vi "Aliasing 1.vi"() -> ()   [LabVIEW 2016]
uses:
  <vilib>/measure/maresamp.llb/Resample Waveform (single shot).vi
  <vilib>/measure/NI_MABase.lvlib
  <vilib>/measure/NI_MAPro.lvlib
panel:
  in  "y-scale [V]":dbl=1.2
  in  "Resolution [Bit]":u8=12
  in  "Sample rate [1/s]":dbl=11.0 min=0.1 step=0.1 format="%.2p"
  in  "Range Volts]":dbl=1.0 format="%0.2p"
  out "Waveform Graph":waveform(dbl)[](graph)=[{"t0"=timestamp(0 s since 1904-01-01), "dt"=0.001, "Y"=array[2000 elements]}, {"t0"=timestamp(0 s since 1904-01-01), "dt"=0.09090909090909091, "Y"=[0.0, -0.5403941761363638, -0.9093128551136365, -0.9895241477272729, -0.755415482954545, -0.2815607244318157, 0.2815607244318157, 0.755415482954545, 0.9895241477272729, 0.9093128551136351, 0.5403941761363593, 0.0, -0.5403941761363593, -0.9093128551136379, -0.9895241477272729, -0.7554154829545403, -0.2815607244318157, 0.2815607244318157, 0.7554154829545497, 0.9895241477272729, 0.9093128551136322, 0.5403941761363593]}, {"t0"=timestamp(0 s since 1904-01-01), "dt"=0.0005, "Y"=array[4000 elements]}]
  in  "Stop":bool
  in  "Signal Type":T1(ring)
  in  "Duty cycle [%]":dbl=50.0
  in  "Phase [deg]":dbl format="%.2p"
  in  "Frequency [Hz]":dbl=10.0 min=0.0 max=100.0 step=0.1 format="%.2p"
  # "Original Wave"
  # "Sampled Wave"
  # "Sampling and Aliasing"
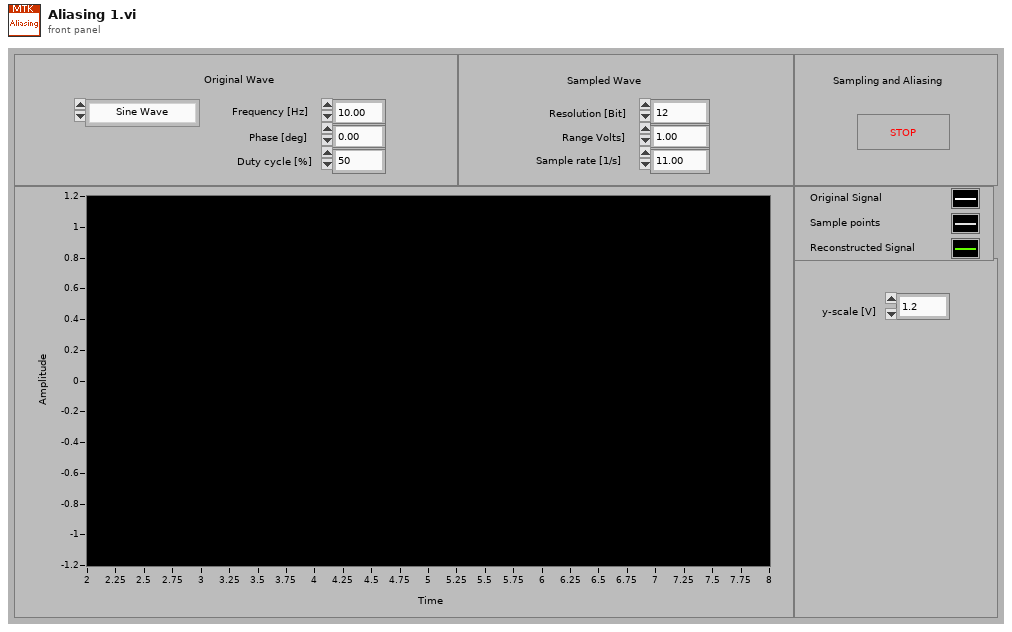
[diagram p1: front panel]
types:
  T1 = enum16{"Sine Wave", "Triangle Wave", "Square Wave", "Sawtooth Wave"}
  T2 = cluster{"Sample rate [1/s]":dbl, "No. of samples":dbl}
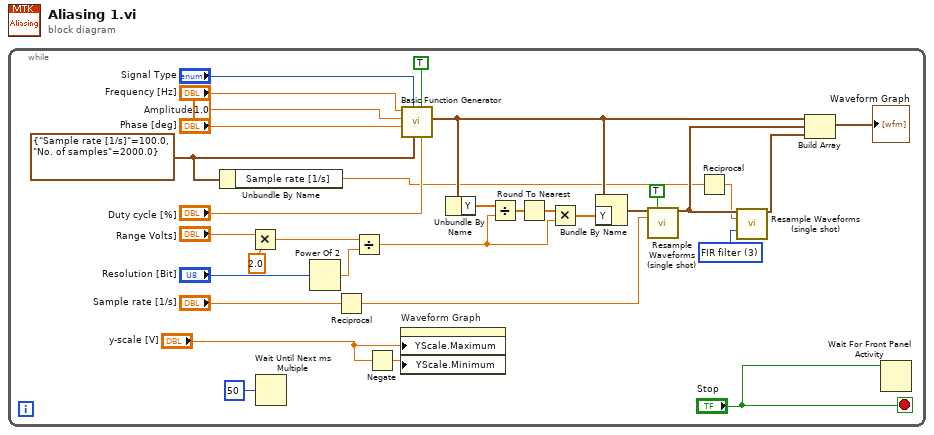
[diagram p0: block diagram]
diagram:
  n1 = while {
    stop <- "Stop" stop-if-true
    w1 = T2 {"Sample rate [1/s]"=100.0, "No. of samples"=2000.0} ("sampling info")
    w4 = u16 3 items=["coerce", "linear", "spline", "FIR filter"] ("interpolation mode")
    w31 = 1.0  # Amplitude
    n2 = Unbundle By Name(w1) -> ("Sample rate [1/s]"=w2:dbl)
    n3 = Multiply(x="Range Volts]", y=2.0) -> (x*y=w22:dbl)
    n4 = Wait Until Next ms Multiple(millisecond multiple=u32 50) -> ()  [unwired: 1 out]
    n5 = Power Of 2(x="Resolution [Bit]") -> (2^x=w24:dbl)
    n6 = Reciprocal(x="Sample rate [1/s]") -> (1/x=w15:dbl)
    n7 = Divide(x=w22, y=w24) -> (x/y=w10:dbl)
    n8 = Negate(x="y-scale [V]") -> (-x=w11:dbl)
    n9 = property on="Waveform Graph" class="WFGraph (strict)"("YScale.Maximum"="y-scale [V]", "YScale.Minimum"=w11) -> ()  [unwired: 2 in, 2 out]
    n10 = call <vilib>:"Basic Function Generator.vi"("square wave duty cycle (%)"="Duty cycle [%]", "reset signal"=TRUE, "sampling info"=w1, "signal type"="Signal Type", "phase"="Phase [deg]", "amplitude"=w31, "frequency"="Frequency [Hz]") -> ("signal out"=w26:waveform(dbl))  [unwired: 2 in, 2 out]
    n11 = Unbundle By Name(w26) -> ("Y"=w20:dbl[])
    n12 = Divide(x=w20, y=w10) -> (x/y=w19:dbl[])
    n13 = Round To Nearest(number=w19) -> (nearest integer value=w18:dbl[])
    n14 = Multiply(x=w18, y=w10) -> (x*y=w21:dbl[])
    n15 = Bundle By Name(cluster=w26, "Y"=w21) -> (w17:waveform(dbl))
    n16 = call-poly <vilib>:"Resample Waveforms (single shot).vi"("waveform in"=w17, "open interval? (F)"=TRUE, "dt"=w15) -> ("resampled waveform out"=w7:waveform(dbl))  [unwired: 4 in, 8 out]
    n17 = Reciprocal(x=w2) -> (1/x=w5:dbl)
    n18 = call-poly <vilib>:"Resample Waveforms (single shot).vi"("waveform in"=w7, "dt"=w5, "interpolation mode"=w4) -> ("resampled waveform out"=w6:waveform(dbl))  [unwired: 4 in, 8 out]
    n19 = Build Array(w26, w7, w6) -> (→"Waveform Graph":waveform(dbl)[])
    n20 = Wait For Front Panel Activity(3:"Stop") -> ()  [unwired: 2 in, 1 out]
  }
